vi "set padding.vi"(8 "error in":errorcluster, 11 "lvlibcrypto digest in":refnum<class "lvlibcrypto cipher.lvclass">) -> (0 "error out":errorcluster, 3 "lvlibcrypto digest out":refnum<class "lvlibcrypto cipher.lvclass">)   [LabVIEW 2016, in "lvlibcrypto cipher.lvclass"]
uses:
  lvlibcrypto cipher.lvclass
  lvlibcrypto cipher.lvclass/lvlibcrypto cipher.ctl
  lv tls dll.lvlib
panel:
  in  "disable padding?":bool
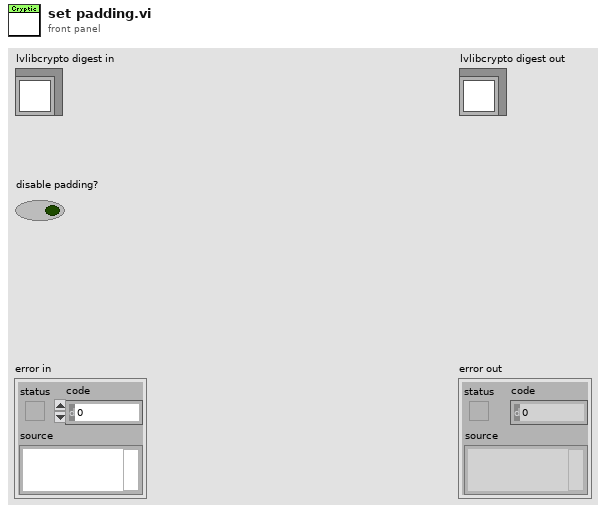
[diagram p1: front panel]
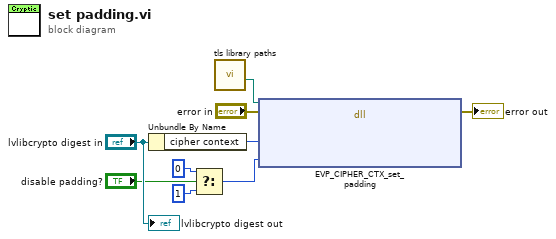
[diagram p0: block diagram]
diagram:
  n1 = Unbundle By Name("lvlibcrypto digest in") -> ("cipher context"=w7:u64)
  n2 = Select(t=0, s="disable padding?", f=1 ("t")) -> (s? t:f=w1:i32)
  n3 = call "tls library paths.vi"() -> ("libcrypto"=w9:path)  [unwired: 8 in, 3 out]
  n4 = dll-call lib="C:/Users/IEUser/Desktop/tlssimple/libcrypto-41.dll" fn="EVP_CIPHER_CTX_set_padding"(path in=w9, error in="error in", "context"=w7, "padding"=w1) -> (error out=→"error out":errorcluster)  [unwired: 4 in, 1 out]
  "lvlibcrypto digest out" <- "lvlibcrypto digest in"
